vi "Destroy Channels.vi"(8 "error in (no error)":errorcluster, 11 "CIFCorePlugin in":refnum<class "CIFCorePlugin.lvclass">) -> (0 "error out":errorcluster, 2 "Unregister Channels":string[](array[string]), 3 "CIFCorePlugin out":refnum<class "CIFCorePlugin.lvclass">)   [LabVIEW 2021, in "CIFCorePlugin.lvclass"]
uses:
  CIFCorePlugin.lvclass
  CIFCorePlugin.lvclass/CIFCorePlugin.ctl
  Channels/CIFChannelMng/CIFChannelMng.lvclass
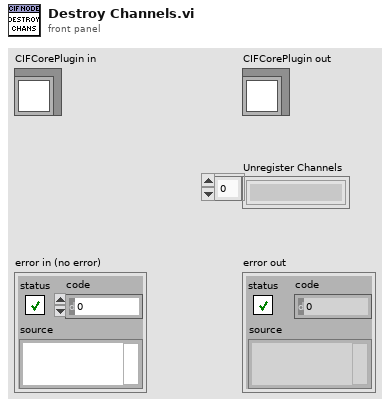
[diagram p1: front panel]
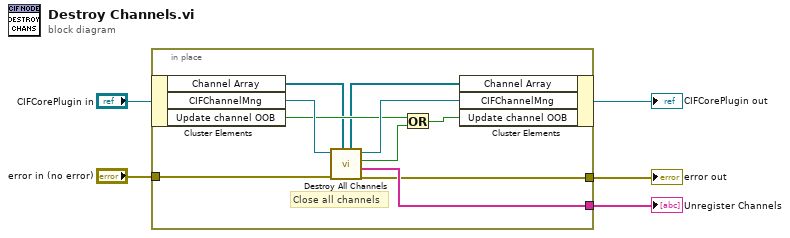
[diagram p0: block diagram]
diagram:
  n1 = in-place {
    in-place-border: "error in (no error)" -> [w7]
    in-place-border: [w6] -> w2
    in-place-border: [w8] -> w1
    # "Close all channels"
    n2 = in-place-cluster #1("CIFCorePlugin in") -> ("Channel Array"=w9:refnum<class "CIFChannels.lvclass">[], "CIFChannelMng"=w15:refnum<class "CIFChannelMng.lvclass">, "Update channel OOB"=w13:bool)
    n3 = call "Destroy All Channels.vi"("Channel Array in"=w9, "error in (no error)"=w7, "CIFChannelMng in"=w15) -> ("error out"=w6:errorcluster, "Unregister Channels"=w8:string[], "Update Channel OOB"=w12:bool, "CIFChannelMng out"=w14:refnum<class "CIFChannelMng.lvclass">, "Channel Array out"=w10:refnum<class "CIFChannels.lvclass">[])  [unwired: 4 in]
    n4 = Or(x=w13, y=w12) -> (x .or. y?=w11:bool)
    n5 = in-place-cluster #1("Channel Array"=w10, "CIFChannelMng"=w14, "Update channel OOB"=w11) -> (→"CIFCorePlugin out":refnum<class "CIFCorePlugin.lvclass">)
  }
  "error out" <- w2
  "Unregister Channels" <- w1
